vi "MergeErrorMessages.vi"(1 "Error Descriptions":string[](array[string]), 2 "Active Errors":bool[](array[boolean])) -> (0 "Merged Error Message":string)   [LabVIEW 2020]
doc: "Merges an array of active error messages into a single error message string."
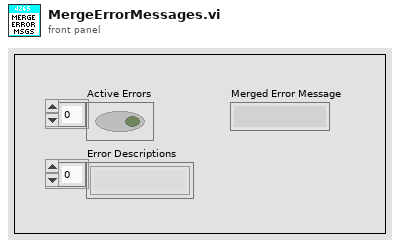
[diagram p1: front panel]
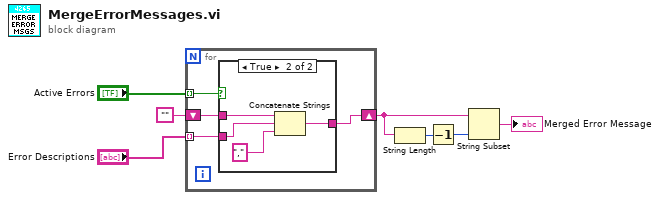
[diagram p0: block diagram]
diagram:
  n1 = for {
    tunnel: "Active Errors" -> [w10] mode=indexing
    shift-right: [w9] -> w2
    shift-left: "" -> [w11]
    tunnel: "Error Descriptions" -> [w8] mode=indexing
    n2 = case shown="True" w10 {
      tunnel: w11 -> [w12 w16]
      tunnel: [w12 w15] -> w9
      tunnel: w8 -> [_ w13]
      frame False {
      }
      frame True {
        n3 = Concatenate Strings(w16, w13, "," ("string")) -> (w15:string)
      }
    }
  }
  n4 = String Length(string=w2) -> (length=w4:i32)
  n5 = Decrement(x=w4) -> (x-1=w3:i32)
  n6 = String Subset(string=w2, length (rest)=w3) -> (substring=→"Merged Error Message":string)  [unwired: 1 in]
